vi "Write U64 Value.vi"(8 "error in (no error)":errorcluster, 10 "U64":u64, 11 "Numeric in":refnum<class "Abs_Double Float.lvclass">) -> (0 "error out":errorcluster, 3 "Numeric out":refnum<class "Abs_Double Float.lvclass">)   [LabVIEW 2021, in "Abs_Double Float.lvclass"]
uses:
  Abs_Double Float.lvclass
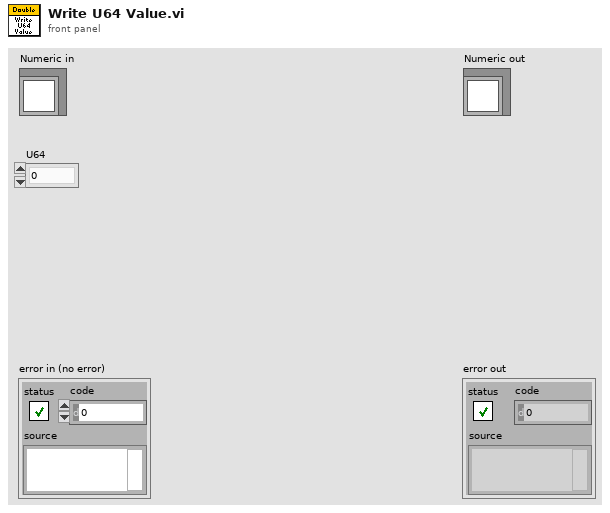
[diagram p1: front panel]
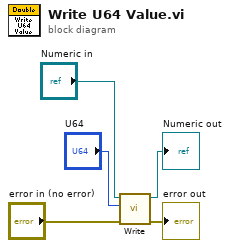
[diagram p0: block diagram]
diagram:
  n1 = call-dynamic "Write.vi"("error in (no error)"="error in (no error)", "Value"="U64", "Double Float.lvclass in"="Numeric in") -> ("error out"=→"error out":errorcluster, "Double Float.lvclass out"=→"Numeric out":refnum<class "Abs_Double Float.lvclass">)  [unwired: 7 in]
